vi "NI9205 Chart.vi"() -> ()   [LabVIEW 2018]
uses:
  <vilib>/Platform/TimedLoop/XDataNode/timing_clust.ctl
  <vilib>/Platform/TimedLoop/XDataNode/nitl_modes.ctl
  <vilib>/Platform/TimedLoop/XDataNode/wakeup.ctl
  <vilib>/Instr/_visa.llb/VISA Configure Serial Port (Instr).vi
  <vilib>/Platform/TimedLoop/XDataNode/loadnilvce.vi
  <vilib>/platform/TimedLoop/XDataNode/XDataNode.xnode
  <vilib>/Platform/TimedLoop/XDataNode/XDNodeRunTimeDep.lvlib
panel:
  in  "Send 2":bool
  in  "Send ESC":bool
  in  "VISA Send Msg":string
  in  "Send":bool
  out "AT Out":string
  out "error out":errorcluster
  in  "error in":errorcluster
  out "Waveform Chart":dbl(graph)
  in  "Stop":bool
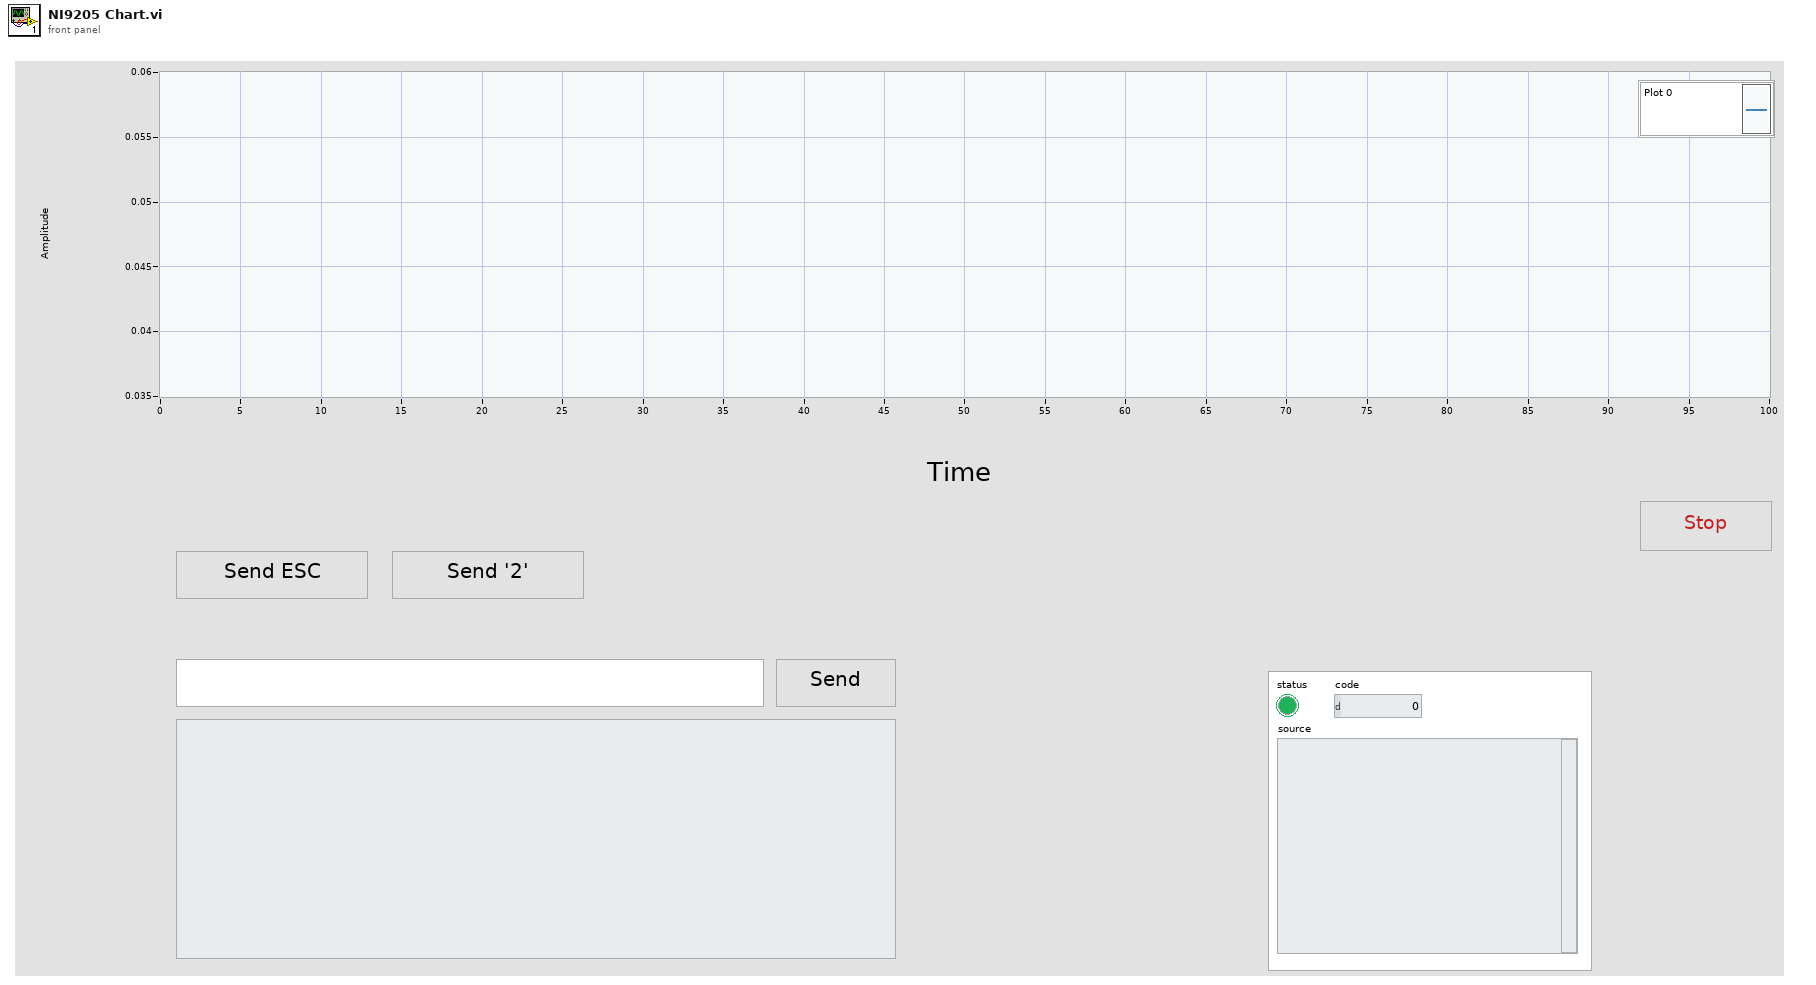
[diagram p1: front panel]
types:
  T1 = typedef "XDNodeRunTimeDep.lvlib/timing_clust.ctl" = cluster{"Expected End [f-1]":u64, "Actual End [f-1]":u64, "Finished Late? [f-1]":bool, "Expected End [i-1]":u64, "Actual End [i-1]":u64, "Finished Late? [i-1]":bool, "Expected Start [i]":u64, "Actual Start [i]":u64, "Expected Start [f]":u64, "Actual Start [f]":u64, "Source Name":string, "Structure Name":string, "Period":i64, "Deadline":i64, "Offset":i64, "Start":i64, "Priority":i32, "Timeout":i32, "Mode":T2, "Wakeup Reason":T3, "Error":errorcluster, "Source Type":string, "Secondary Source Type":string, "Global End Time":u64, "Global Start Time":u64, "Frame Duration":u64, "Iteration Duration":u64, "Assigned CPU":i32, "I/O Scan Engine Mode":u32}
  T2 = typedef "XDNodeRunTimeDep.lvlib/nitl_modes.ctl" = enum32{"No Change", "Process missed periods, maintain original phase", "Discard missed periods, maintain original phase", "Process missed periods, ignore original phase", "Discard missed periods, ignore original phase"}
  T3 = typedef "XDNodeRunTimeDep.lvlib/wakeup.ctl" = enum32{"Normal", "Aborted", "Asynchronous wakeup", "Timing source error", "Timed loop error", "Timeout"}
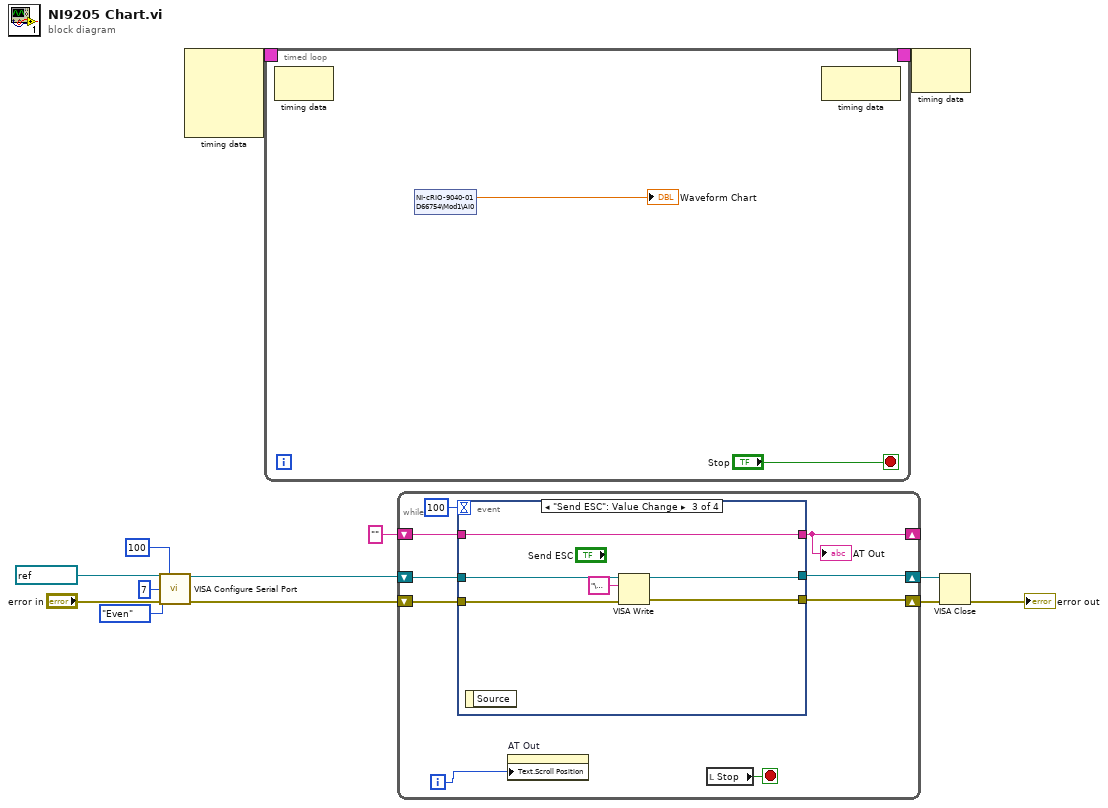
[diagram p0: block diagram]
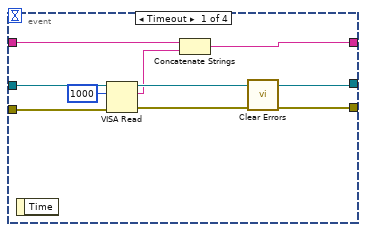
[diagram p2: hidden frame]
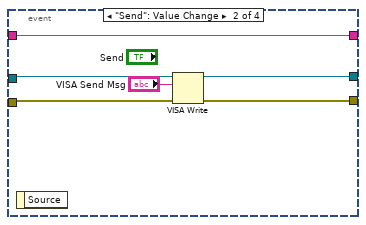
[diagram p3: hidden frame]
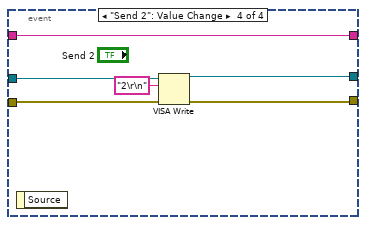
[diagram p4: hidden frame]
diagram:
  n1 = call-poly "VISA Configure Serial Port"("VISA resource name"=refnum<visa-resource-name> "COM1", "timeout (10sec)"=u32 100, "data bits (8)"=u16 7, "parity (0:none)"=enum16{"None", "Odd", "Even", "Mark", "Space"}."Even", "error in (no error)"="error in") -> ("VISA resource name out"=w11:refnum<visa-resource-name>, "error out"=w10:errorcluster)  [unwired: 9 in]
  n2 = node-c288() -> (w13:T1)  [unwired: 4 in]
  n3 = timed-loop {
    timing: w13 -> [_]
    timing-out: [_] -> w12
    stop <- "Stop" stop-if-true
    n4 = node-c288() -> ()  [unwired: 1 in, 1 out]
    n5 = shared-variable "NI-cRIO-9040-01D66754\\Mod1\\AI0"() -> (→"Waveform Chart":dbl)  [unwired: 1 in, 1 out]
    n6 = node-c288() -> ()  [unwired: 1 in, 1 out]
  }
  n7 = while {
    shift-right: [w22] -> w7
    shift-left: w10 -> [w23]
    shift-right: [w18] -> _
    shift-left: "" -> [w19]
    shift-right: [w21] -> w8
    shift-left: w11 -> [w24]
    i -> [w25]
    stop <- w26 stop-if-true
    n8 = event shown="[2] \"Send ESC\": Value Change" {
      selector: _ -> [_ _ _ _]
      dyn-events: _ -> [_ _ _ _]
      timeout: 100 -> [_ _ _ _]
      tunnel: w24 -> [w34 w41 w45 w52]
      tunnel: w23 -> [w35 w40 w46 w51]
      tunnel: [w31 w39 w43 w50] -> w22
      tunnel: [w33 w38 w44 w49] -> w21
      tunnel: w19 -> [w29 w36 w47 w53]
      tunnel: [w28 w36 w47 w53] -> w18
      event Timeout {
        n9 = event-data() -> ()  [unwired: 1 in, 1 out]
        n10 = VISA Read(VISA resource name=w34, byte count=u32 1000, error in (no error)=w35) -> (VISA resource name out=w33:refnum<visa-resource-name>, read buffer=w30:string, error out=w32:errorcluster)  [unwired: 1 out]
        n11 = Concatenate Strings(w29, w30) -> (w28:string)
        n12 = call <vilib>:"Clear Errors.vi"("error in (no error)"=w32) -> ("error out"=w31:errorcluster)  [unwired: 5 in, 1 out]
      }
      event "Send": Value Change {
        n13 = event-data() -> ()  [unwired: 1 in, 1 out]
        n14 = VISA Write(VISA resource name=w41, write buffer="VISA Send Msg", error in (no error)=w40) -> (VISA resource name out=w38:refnum<visa-resource-name>, error out=w39:errorcluster)  [unwired: 1 out]
      }
      event "Send ESC": Value Change {
        n15 = event-data() -> ()  [unwired: 1 in, 1 out]
        n16 = VISA Write(VISA resource name=w45, write buffer="\u001b", error in (no error)=w46) -> (VISA resource name out=w44:refnum<visa-resource-name>, error out=w43:errorcluster)  [unwired: 1 out]
      }
      event "Send 2": Value Change {
        n17 = event-data() -> ()  [unwired: 1 in, 1 out]
        n18 = VISA Write(VISA resource name=w52, write buffer="2\r\n", error in (no error)=w51) -> (VISA resource name out=w49:refnum<visa-resource-name>, error out=w50:errorcluster)  [unwired: 1 out]
      }
    }
    "AT Out" <- w18
    n19 = property on="AT Out" class="Str"("Text.Scroll Position"=w25) -> ()  [unwired: 2 in, 2 out]
    n20 = local read "Stop"() -> (w26:bool)
  }
  n21 = node-c288(w12) -> ()  [unwired: 1 out]
  n22 = VISA Close(VISA resource name=w8, error in (no error)=w7) -> (error out=→"error out":errorcluster)
